vi "Create Stop Event After Fault.vi"(8 "error in":errorcluster, 11 "user event datatype":string) -> (0 "error out":errorcluster, 3 "user event":refnum<user-event>)   [LabVIEW 2026]
doc: "Create the controller shutdown user event even when initialization failed. Return the original initialization error first, then event-creation error. No retry, wait or dialog. Input event data defines a string user event; output event is owned by the controller core and must be destroyed after its parallel loop joins."
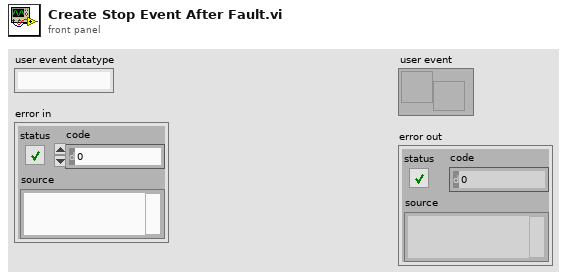
[diagram p1: front panel]
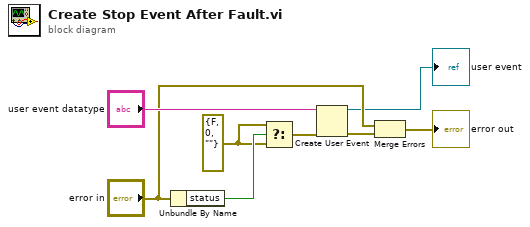
[diagram p0: block diagram]
diagram:
  w7 = errorcluster {"status"=FALSE, "code"=0, "source"=""}
  n1 = Unbundle By Name("error in") -> ("status"=w8:bool)
  n2 = Select(t=w7, s=w8, f=w7) -> (s? t:f=w5:errorcluster)
  n3 = Create User Event(user event datatype="user event datatype", error in=w5) -> (user event=→"user event":refnum<user-event>, error out=w3:errorcluster)
  n4 = Merge Errors("error in", w3) -> (→"error out":errorcluster)
